vi "ReadViRef.vi"(8 "error in (no error)":errorcluster caption="错误输入（无错误）", 11 "ChartView Worker 输入":refnum<class "ChartView Worker.lvclass">) -> (0 "error out":errorcluster caption="错误输出", 2 "VI":refnum<vi>, 3 "ChartView Worker 输出":refnum<class "ChartView Worker.lvclass">)   [LabVIEW 2018, in "ChartView Worker.lvclass"]
uses:
  ChartView Worker.lvclass
  ChartView Worker.lvclass/ChartView Worker.ctl
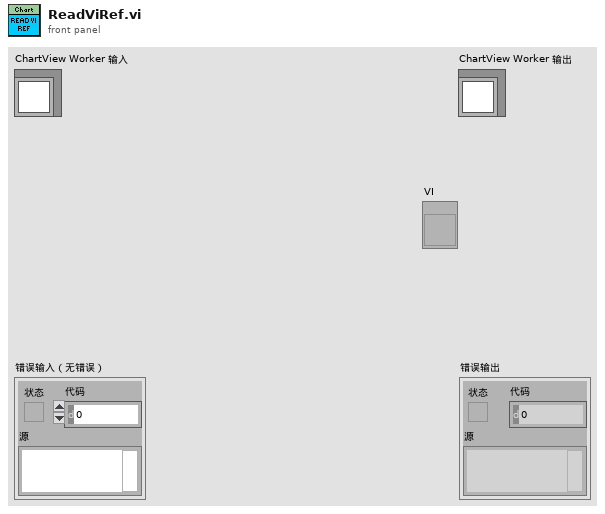
[diagram p1: front panel]
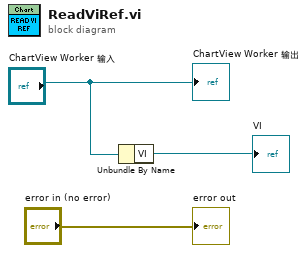
[diagram p0: block diagram]
diagram:
  n1 = Unbundle By Name("ChartView Worker 输入") -> ("VI"=→"VI":refnum<vi>)
  "error out" <- "error in (no error)"
  "ChartView Worker 输出" <- "ChartView Worker 输入"
